vi "Create FP Control Indices Map.vi"(8 "error in":errorcluster, 11 "Frontpanel Ref in":refnum<vi>) -> (0 "error out":errorcluster, 2 "Control Idxs":map{string, i32}(c390), 3 "Frontpanel Ref out":refnum<vi>)   [LabVIEW 2019, in "UI Actor.lvlib" / "UI Actor.lvclass"]
uses:
  UI Actor.lvclass
  UI Actor.lvclass/UI Actor.ctl
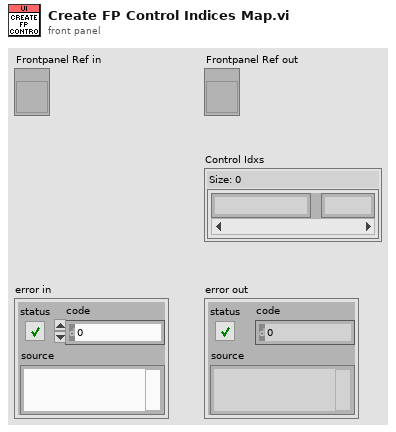
[diagram p1: front panel]
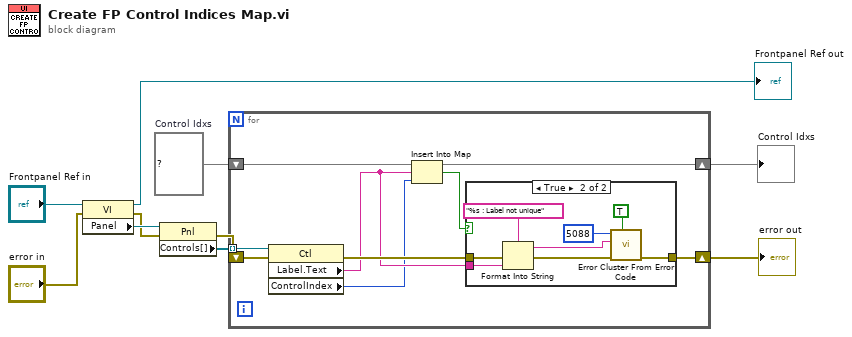
[diagram p0: block diagram]
diagram:
  w6 = map{string, i32} {}  # Control Idxs
  n1 = property class="VI"(reference="Frontpanel Ref in", error in="error in") -> (reference out=→"Frontpanel Ref out":refnum<vi>, error out=w2:errorcluster, "Panel"=w10:refnum<vi>)
  n2 = property class="Pnl"(reference=w10, error in=w2) -> (error out=w7:errorcluster, "Controls[]"=w8:refnum<vi>[])  [unwired: 1 out]
  n3 = for {
    tunnel: w8 -> [w19] mode=indexing
    shift-right: [w16] -> w1
    shift-left: w6 -> [w18]
    shift-right: [w12] -> w5
    shift-left: w7 -> [w17]
    n4 = property class="Ctl"(reference=w19, error in=w17) -> (error out=w15:errorcluster, "Label.Text"=w14:string, "ControlIndex"=w11:i32)  [unwired: 1 out]
    n5 = Insert Into Map(map in=w18, key=w14, value=w11) -> (map out=w16:map{string, i32}, key already included?=w13:bool)  [unwired: 1 out]
    n6 = case shown="True" w13 {
      tunnel: w15 -> [w20 w28]
      tunnel: w14 -> [_ w26]
      tunnel: [w20 w21] -> w12
      frame False {
      }
      frame True {
        n7 = Format Into String(format string="%s : Label not unique", error in=w28, w26) -> (resulting string=w23:string, error out=w24:errorcluster)  [unwired: 1 in]
        n8 = call <vilib>:"Error Cluster From Error Code.vi"("show call chain? (False)"=TRUE, "error in (no error)"=w24, "error message (\"\")"=w23, "error code (0)"=5088) -> ("error out"=w21:errorcluster)  [unwired: 5 in]
      }
    }
  }
  "error out" <- w5
  "Control Idxs" <- w1
